vi "frameratetest_mono12.vi"() -> ()   [LabVIEW 2019]
panel:
  out "Software FPS":dbl
  out "Camera FPS":dbl
  out "Image":u16[][](graph)
  out "Camera Serial":string
  out "Camera Version":string
  out "Camera Model":string
  out "SMD":dbl
  in  "Scan Mode":dbl min=0.0 max=0.0
  in  "Exposure":dbl min=0.0 max=0.0
  out "EXP":dbl
  out "SVW":i32
  out "SHW":i32
  out "SVO":i32
  out "SHO":i32
  in  "V Width":i32 min=0 max=0
  in  "V Offset":i32 min=0 max=0
  in  "H Width":i32 min=0 max=0
  in  "H Offset":i32 min=0 max=0
  in  "Binning":u16(ring)=1 items=["1x1"=1, "2x2"=2, "4x4"=4]
  out "Elapsed Time":u32
  out "Total Frames":i32
  in  "Display":bool=TRUE
  out "error out":errorcluster
  in  "stop":bool
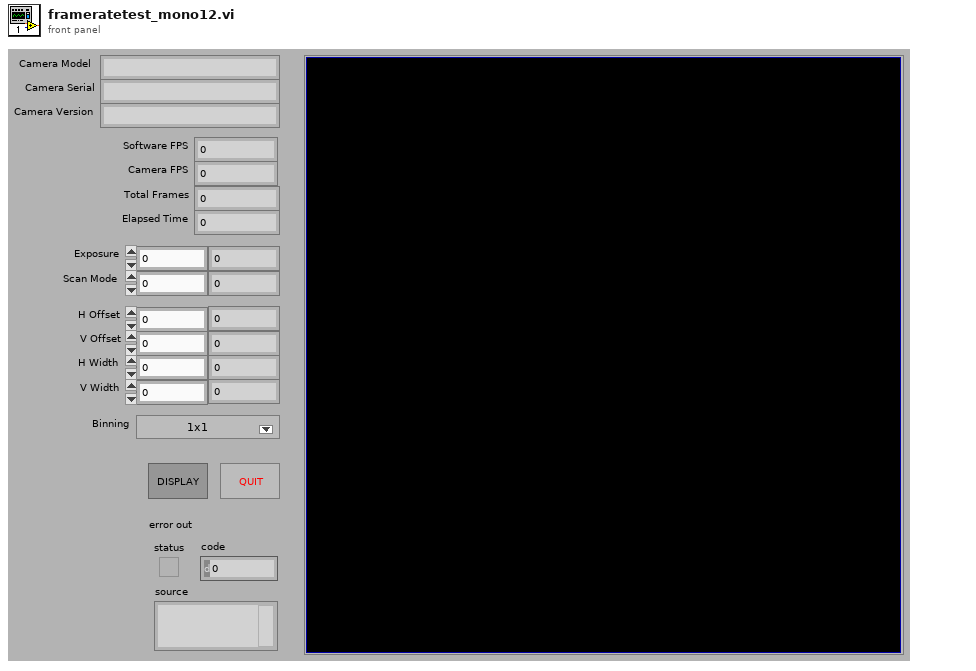
[diagram p1: front panel]
types:
  T1 = cluster{"Model":string, "Camera ID":string, "Firmware":string}
  T2 = typedef "LVMinMaxIncTypeDef.ctl" = cluster{"Minimum":dbl, "Maximum":dbl, "Increment":dbl}
  T3 = cluster{"H Offset":cluster{"Value":i32, "Limits":T2}, "V Offset":cluster{"Value":i32, "Limits":T2}, "H Size":cluster{"Value":i32, "Limits":T2}, "V Size":cluster{"Value":i32, "Limits":T2}}
  T4 = cluster{"H Offset":i32, "V Offset":i32, "H Width":i32, "V Width":i32}
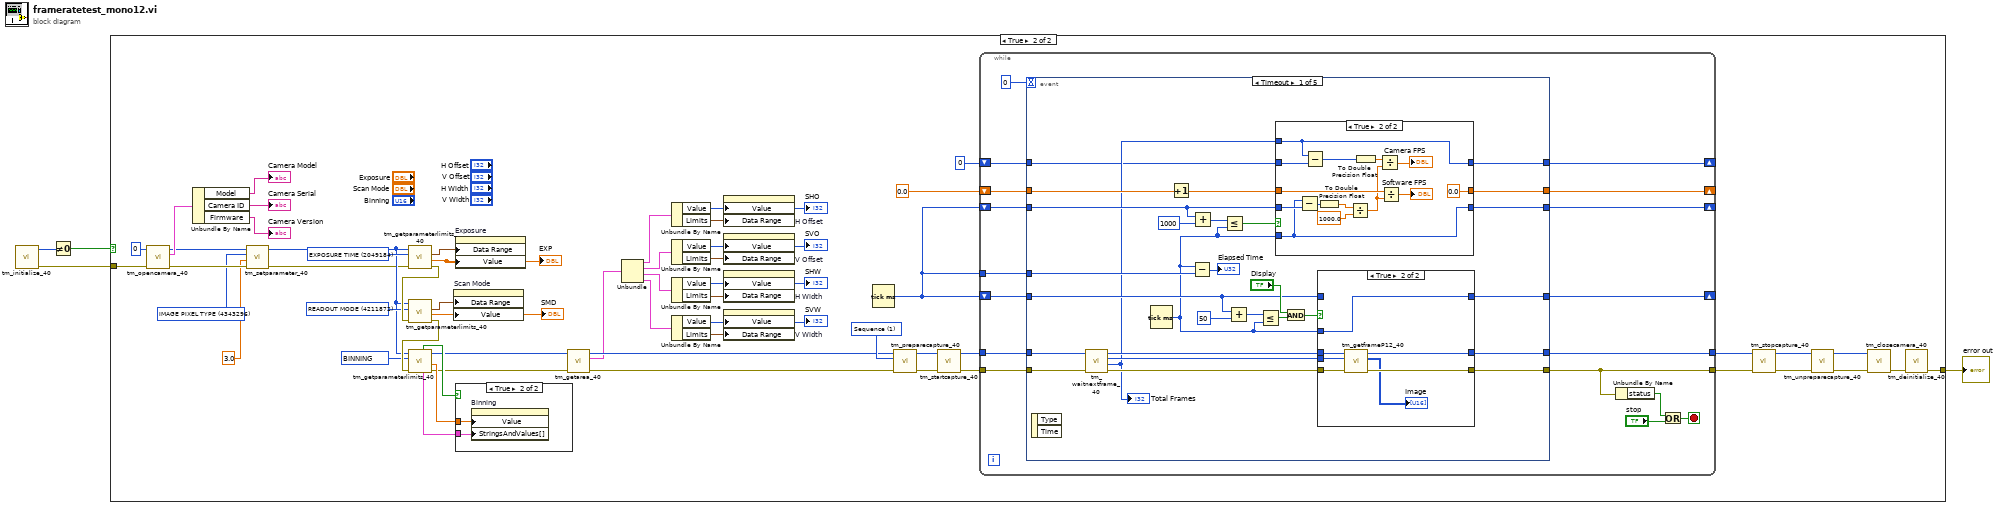
[diagram p0: block diagram]
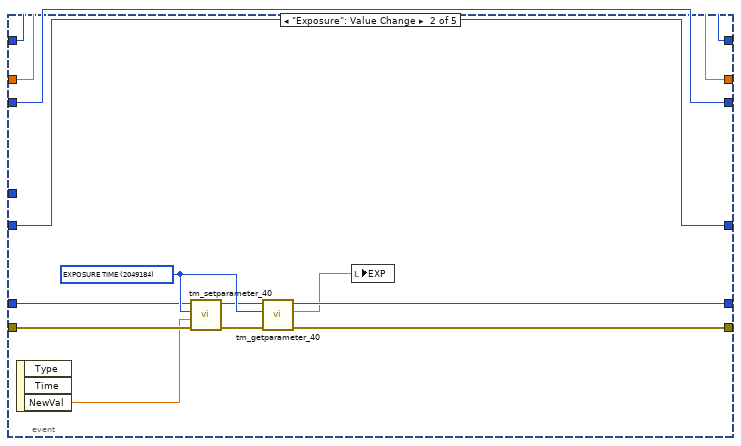
[diagram p6: hidden frame]
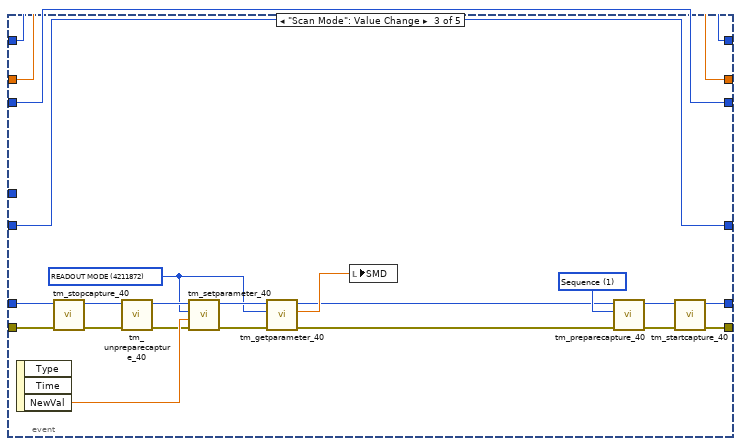
[diagram p7: hidden frame]
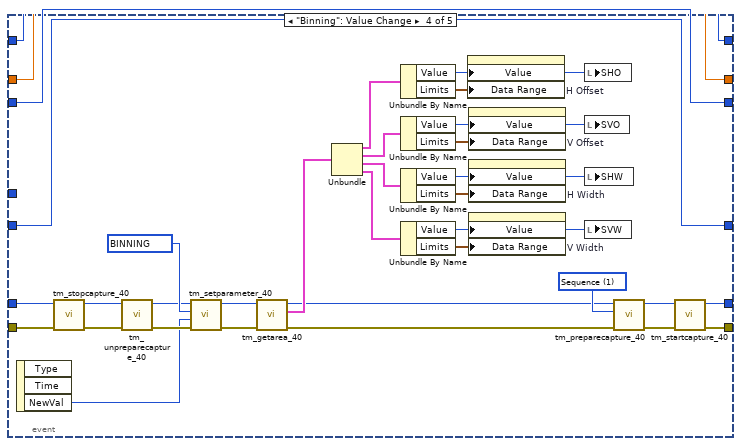
[diagram p8: hidden frame]
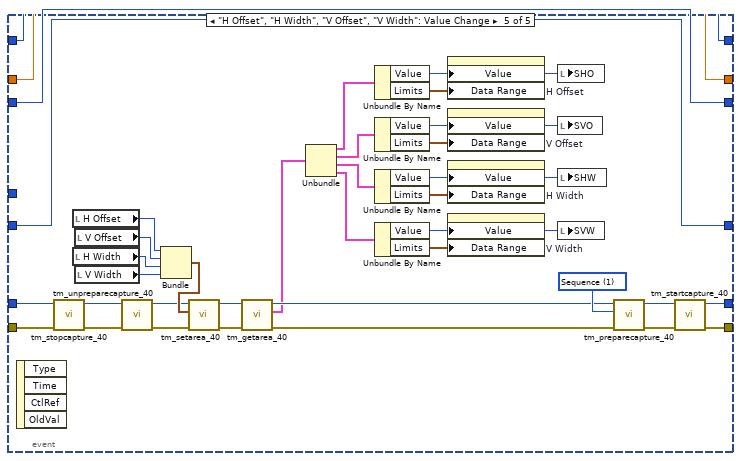
[diagram p9: hidden frame]
diagram:
  n1 = call <userlib>:"tm_initialize_40.vi"() -> ("error out"=w2:errorcluster, "Number Of Cameras"=w1:u32)  [unwired: 8 in, 2 out]
  n2 = Not Equal To 0?(x=w1) -> (x != 0?=w4:bool)
  n3 = case shown="True" w4 {
    tunnel: [w5 w59] -> w3
    tunnel: w2 -> [w5 w62]
    frame False {
    }
    frame True {
      w7 = u32 4343296 items=["SENSOR MODE"=4212128, "READOUT SPEED"=4211872, "READOUT DIRECTION"=4211904, "BIT PER CHANNEL"=4342976, "TRIGGER GLOBAL EXPOSURE"=2049680, "TRIGGER DELAY"=1066480, "INTERNAL TRIGGER HANDLING"=1066496, "SENSOR TEMPERATURE"=2115232, "SENSOR COOLER STATUS"=2115280, "EXPOSURE TIME"=2049184, "DEFECT CORRECT MODE"=4670368, "HOT PIXEL CORRECT LEVEL"=4670400, "BINNING"=4215968, "TIMING READOUT TIME"=4223904, "INTERNAL FRAME RATE"=4225952, "INTERNAL FRAME INTERVAL"=4225968, "INTERNAL LINE SPEED"=4226000, "INTERNAL LINE INTERVAL"=4226016, "IMAGE WIDTH"=4343200, "IMAGE HEIGHT"=4343216, "IMAGE ROWBYTES"=4343232, "IMAGE FRAMEBYTES"=4343248, "IMAGE PIXEL TYPE"=4343296, "NUMBER OF OUTPUT TRIGGER CONNECTOR"=1852320, "OUTPUT TRIGGER SOURCE[0]"=1852576, "OUTPUT TRIGGER SOURCE[1]"=1852832, "OUTPUT TRIGGER SOURCE[2]"=1853088, "OUTPUT TRIGGER POLARITY[0]"=1852592, "OUTPUT TRIGGER POLARITY[1]"=1852848, "OUTPUT TRIGGER POLARITY[2]"=1853104, "OUTPUT TRIGGER ACTIVE[0]"=1852608, "OUTPUT TRIGGER ACTIVE[1]"=1852864, "OUTPUT TRIGGER ACTIVE[2]"=1853120, "OUTPUT TRIGGER DELAY[0]"=1852624, "OUTPUT TRIGGER DELAY[1]"=1852880, "OUTPUT TRIGGER DELAY[2]"=1853136, "OUTPUT TRIGGER PERIOD[0]"=1852640, "OUTPUT TRIGGER PERIOD[1]"=1852896, "OUTPUT TRIGGER PERIOD[2]"=1853152, "OUTPUT TRIGGER KIND[0]"=1852656, "OUTPUT TRIGGER KIND[1]"=1852912, "OUTPUT TRIGGER KIND[2]"=1853168, "OUTPUT TRIGGER BASE SENSOR[0]"=1852672, "OUTPUT TRIGGER BASE SENSOR[1]"=1852928, "OUTPUT TRIGGER BASE SENSOR[2]"=1853184, "OUTPUT TRIGGER PRE HSYNC COUNT"=1852704] ("Parameter")
      w33 = u32 2049184 items=["BINNING"=4215968, "BITS PER CHANNEL"=4342976, "ACTIVE VIEW INDEX"=4343136, "CCD MODE"=4212384, "SENSOR MODE"=4212128, "READOUT MODE"=4211872, "EXPOSURE TIME"=2049184, "CONTRAST GAIN"=3163312, "CONTRAST OFFSET"=3163328, "LIGHT MODE"=2114720, "SENSITIVITY"=2114992, "WHITE BALANCE"=3163568, "PHOTON IMAGING MODE"=2115200, "HIGH DYNAMIC RANGE MODE"=3163360, "TRIGGER SOURCE"=1066144, "TRIGGER ACTIVE"=1066160, "TRIGGER MODE"=1066400, "TRIGGER POLARITY"=1066416, "TRIGGER GLOBAL EXPOSURE"=2049680, "FIRST TRIGGER BEHAVIOR"=2049696, "TRIGGER TIMES"=1066448, "OUTPUT TRIGGER POLARITY"=1852592, "OUTPUT TRIGGER DELAY"=1852624, "OUTPUT TRIGGER PERIOD"=1852640, "TEMPERATURE"=2115232, "TEMPERATURE TARGET"=2115264, "SENSOR COOLER FAN"=2115296, "MECHANICAL SHUTTER"=2115488, "BACK FOCUS POSITION"=8422304, "FRAMEBUNDLE MODE"=4346784, "FRAMEBUNDLE NUMBER"=4346800, "LINEBUNDLE HEIGHT"=4212192, "TRIGGER CONNECTOR"=1066432, "IMAGE PIXEL TYPE"=4343296, "OUTPUT TRIGGER KIND"=1852656, "READOUT DIRECTION"=4211904, "CHANNEL SYNC"=1852352] ("Parameter")
      w34 = u32 4211872 items=["BINNING"=4215968, "BITS PER CHANNEL"=4342976, "ACTIVE VIEW INDEX"=4343136, "CCD MODE"=4212384, "SENSOR MODE"=4212128, "READOUT MODE"=4211872, "EXPOSURE TIME"=2049184, "CONTRAST GAIN"=3163312, "CONTRAST OFFSET"=3163328, "LIGHT MODE"=2114720, "SENSITIVITY"=2114992, "WHITE BALANCE"=3163568, "PHOTON IMAGING MODE"=2115200, "HIGH DYNAMIC RANGE MODE"=3163360, "TRIGGER SOURCE"=1066144, "TRIGGER ACTIVE"=1066160, "TRIGGER MODE"=1066400, "TRIGGER POLARITY"=1066416, "TRIGGER GLOBAL EXPOSURE"=2049680, "FIRST TRIGGER BEHAVIOR"=2049696, "TRIGGER TIMES"=1066448, "OUTPUT TRIGGER POLARITY"=1852592, "OUTPUT TRIGGER DELAY"=1852624, "OUTPUT TRIGGER PERIOD"=1852640, "TEMPERATURE"=2115232, "TEMPERATURE TARGET"=2115264, "SENSOR COOLER FAN"=2115296, "MECHANICAL SHUTTER"=2115488, "BACK FOCUS POSITION"=8422304, "FRAMEBUNDLE MODE"=4346784, "FRAMEBUNDLE NUMBER"=4346800, "LINEBUNDLE HEIGHT"=4212192, "TRIGGER CONNECTOR"=1066432, "IMAGE PIXEL TYPE"=4343296, "OUTPUT TRIGGER KIND"=1852656, "READOUT DIRECTION"=4211904, "CHANNEL SYNC"=1852352] ("Parameter")
      w35 = u32 4215968 items=["BINNING"=4215968, "BITS PER CHANNEL"=4342976, "ACTIVE VIEW INDEX"=4343136, "CCD MODE"=4212384, "SENSOR MODE"=4212128, "READOUT MODE"=4211872, "EXPOSURE TIME"=2049184, "CONTRAST GAIN"=3163312, "CONTRAST OFFSET"=3163328, "LIGHT MODE"=2114720, "SENSITIVITY"=2114992, "WHITE BALANCE"=3163568, "PHOTON IMAGING MODE"=2115200, "HIGH DYNAMIC RANGE MODE"=3163360, "TRIGGER SOURCE"=1066144, "TRIGGER ACTIVE"=1066160, "TRIGGER MODE"=1066400, "TRIGGER POLARITY"=1066416, "TRIGGER GLOBAL EXPOSURE"=2049680, "FIRST TRIGGER BEHAVIOR"=2049696, "TRIGGER TIMES"=1066448, "OUTPUT TRIGGER POLARITY"=1852592, "OUTPUT TRIGGER DELAY"=1852624, "OUTPUT TRIGGER PERIOD"=1852640, "TEMPERATURE"=2115232, "TEMPERATURE TARGET"=2115264, "SENSOR COOLER FAN"=2115296, "MECHANICAL SHUTTER"=2115488, "BACK FOCUS POSITION"=8422304, "FRAMEBUNDLE MODE"=4346784, "FRAMEBUNDLE NUMBER"=4346800, "LINEBUNDLE HEIGHT"=4212192, "TRIGGER CONNECTOR"=1066432, "IMAGE PIXEL TYPE"=4343296, "OUTPUT TRIGGER KIND"=1852656, "READOUT DIRECTION"=4211904, "CHANNEL SYNC"=1852352] ("Parameter")
      w57 = 1 items=["Snap", "Sequence"] ("Capture mode")
      n4 = call <userlib>:"tm_opencamera_40.vi"("error in (no error)"=w62, "Camera Index"=u32 0) -> ("error out"=w11:errorcluster, "Camera Details"=w44:T1, "Handle out"=w10:u32)  [unwired: 7 in]
      n5 = Unbundle By Name(w44) -> ("Model"=→"Camera Model":string, "Camera ID"=→"Camera Serial":string, "Firmware"=→"Camera Version":string)
      n6 = call <userlib>:"tm_setparameter_40.vi"("error in (no error)"=w11, "Value in"=3.0, "Parameter"=w7, "Handle in"=w10) -> ("error out"=w8:errorcluster, "Handle out"=w9:u32)  [unwired: 6 in]
      n7 = call <userlib>:"tm_getparameterlimits_40.vi"("error in (no error)"=w8, "Parameter"=w33, "Handle in"=w9) -> ("error out"=w40:errorcluster, "default"=w25:dbl, "Range"=w26:cluster{"min":dbl, "max":dbl, "step":dbl})  [unwired: 2 in, 4 out]
      "EXP" <- w25
      n8 = call <userlib>:"tm_getparameterlimits_40.vi"("error in (no error)"=w40, "Parameter"=w34, "Handle in"=w9) -> ("error out"=w39:errorcluster, "default"=w27:dbl, "Range"=w28:cluster{"min":dbl, "max":dbl, "step":dbl})  [unwired: 2 in, 4 out]
      "SMD" <- w27
      n9 = call <userlib>:"tm_getparameterlimits_40.vi"("error in (no error)"=w39, "Parameter"=w35, "Handle in"=w9) -> ("error out"=w32:errorcluster, "default"=w37:dbl, "Handle out"=w31:u32, "Value Names"=w36:cluster{"Name":string, "Value":dbl}[], "Writable"=w38:bool)  [unwired: 2 in, 2 out]
      n10 = property on="Scan Mode" class="DigNum (strict)"("Data Range"=w28, "Value"=w27) -> ()  [unwired: 2 in, 2 out]
      n11 = property on="Exposure" class="DigNum (strict)"("Data Range"=w26, "Value"=w25) -> ()  [unwired: 2 in, 2 out]
      n12 = case shown="True" w38 {
        tunnel: w36 -> [_ w64]
        tunnel: w37 -> [_ w63]
        frame False {
        }
        frame True {
          n13 = property on="Binning" class="Ring (strict)"("Value"=w63, "StringsAndValues[]"=w64) -> ()  [unwired: 2 in, 2 out]
        }
      }
      n14 = call <userlib>:"tm_getarea_40.vi"("error in (no error)"=w32, "Handle in"=w31) -> ("error out"=w30:errorcluster, "Sub Region"=w20:T3, "Handle out"=w29:u32)  [unwired: 7 in]
      n15 = Unbundle(w20) -> ("H Offset"=w24:cluster{"Value":i32, "Limits":T2}, "V Offset"=w23:cluster{"Value":i32, "Limits":T2}, "H Size"=w22:cluster{"Value":i32, "Limits":T2}, "V Size"=w21:cluster{"Value":i32, "Limits":T2})
      n16 = Unbundle By Name(w24) -> ("Value"=w19:i32, "Limits"=w18:T2)
      "SHO" <- w19
      n17 = Unbundle By Name(w23) -> ("Value"=w13:i32, "Limits"=w12:T2)
      "SVO" <- w13
      n18 = Unbundle By Name(w22) -> ("Value"=w15:i32, "Limits"=w14:T2)
      "SHW" <- w15
      n19 = Unbundle By Name(w21) -> ("Value"=w17:i32, "Limits"=w16:T2)
      "SVW" <- w17
      n20 = property on="H Offset" class="DigNum (strict)"("Value"=w19, "Data Range"=w18) -> ()  [unwired: 2 in, 2 out]
      n21 = property on="V Offset" class="DigNum (strict)"("Value"=w13, "Data Range"=w12) -> ()  [unwired: 2 in, 2 out]
      n22 = property on="H Width" class="DigNum (strict)"("Value"=w15, "Data Range"=w14) -> ()  [unwired: 2 in, 2 out]
      n23 = property on="V Width" class="DigNum (strict)"("Value"=w17, "Data Range"=w16) -> ()  [unwired: 2 in, 2 out]
      n24 = Tick Count (ms)() -> (millisecond timer value=w52:u32)
      n25 = call <userlib>:"tm_preparecapture_40.vi"("error in (no error)"=w30, "Capture mode"=w57, "Handle in"=w29) -> ("error out"=w55:errorcluster, "Handle out"=w56:u32)  [unwired: 5 in, 2 out]
      n26 = call <userlib>:"tm_startcapture_40.vi"("error in (no error)"=w55, "Handle in"=w56) -> ("error out"=w54:errorcluster, "Handle out"=w53:u32)  [unwired: 8 in]
      n27 = while {
        tunnel: w54 -> [w71]
        tunnel: [w69] -> w51
        tunnel: [w68] -> w50
        shift-right: [w77] -> _
        shift-left: w52 -> [w75]
        shift-right: [w78] -> _
        shift-left: 0.0 -> [w76]
        shift-right: [w70] -> _
        shift-left: w52 -> [w73]
        tunnel: w53 -> [w72]
        tunnel: w52 -> [w74]
        shift-right: [w65] -> _
        shift-left: 0 -> [w66]
        stop <- w79 stop-if-true
        n28 = event shown="[0] Timeout" {
          selector: _ -> [_ _ _ _ _]
          dyn-events: _ -> [_ _ _ _ _]
          timeout: 0 -> [_ _ _ _ _]
          tunnel: [w86 w147 w169 w198 w235] -> w78
          tunnel: [w85 w148 w170 w199 w236] -> w77
          tunnel: w76 -> [w95 w147 w169 w198 w235]
          tunnel: w75 -> [w88 w148 w170 w199 w236]
          tunnel: w74 -> [w91 _ _ _ _]
          tunnel: w73 -> [w96 w149 w171 w205 w242]
          tunnel: w72 -> [w98 w142 w166 w197 w229]
          tunnel: w71 -> [w97 w144 w165 w196 w228]
          tunnel: [w94 w149 w171 w205 w242] -> w70
          tunnel: [w93 w139 w160 w200 w237] -> w69
          tunnel: [w92 w137 w161 w201 w238] -> w68
          tunnel: w66 -> [w83 w146 w159 w193 w223]
          tunnel: [w82 w146 w159 w193 w223] -> w65
          event Timeout {
            n29 = event-data() -> ()  [unwired: 1 in, 2 out]
            n30 = call <userlib>:"tm_waitnextframe_40.vi"("error in (no error)"=w97, "Handle in"=w98) -> ("error out"=w102:errorcluster, "Frame Count"=w84:i32, "Frame Index"=w101:i32, "Handle out"=w103:u32)  [unwired: 6 in]
            "Total Frames" <- w84
            n31 = Tick Count (ms)() -> (millisecond timer value=w90:u32)
            n32 = Increment(x=w95) -> (x+1=w87:dbl)
            n33 = Subtract(x=w90, y=w91) -> (x-y=→"Elapsed Time":u32)
            n34 = Add(x=w88, y=u32 1000) -> (x+y=w109:u32)
            n35 = Less Or Equal?(x=w109, y=w90) -> (x <= y?=w89:bool)
            n36 = Add(x=w96, y=u32 50) -> (x+y=w107:u32)
            n37 = Less Or Equal?(x=w107, y=w90) -> (x <= y?=w105:bool)
            n38 = case shown="True" w89 {
              tunnel: w88 -> [w112 w121]
              tunnel: [w112 w118] -> w85
              tunnel: w87 -> [w111 w124]
              tunnel: w90 -> [_ w118]
              tunnel: [w111 0.0] -> w86
              tunnel: w84 -> [_ w113]
              tunnel: w83 -> [w110 w116]
              tunnel: [w110 w113] -> w82
              frame False {
              }
              frame True {
                n39 = Subtract(x=w118, y=w121) -> (x-y=w120:u32)
                n40 = Subtract(x=w113, y=w116) -> (x-y=w114:i32)
                n41 = To Double Precision Float(number=w120) -> (double precision float=w126:dbl)
                n42 = Divide(x=w126, y=1000.0) -> (x/y=w117:dbl)
                n43 = To Double Precision Float(number=w114) -> (double precision float=w115:dbl)
                n44 = Divide(x=w115, y=w117) -> (x/y=→"Camera FPS":dbl)
                n45 = Divide(x=w124, y=w117) -> (x/y=→"Software FPS":dbl)
              }
            }
            n46 = And(x="Display", y=w105) -> (x .and. y?=w100:bool)
            n47 = case shown="True" w100 {
              tunnel: w96 -> [w129 _]
              tunnel: w90 -> [_ w136]
              tunnel: [w129 w136] -> w94
              tunnel: w103 -> [w128 w135]
              tunnel: w102 -> [w127 w134]
              tunnel: [w128 w133] -> w93
              tunnel: [w127 w132] -> w92
              tunnel: w101 -> [_ w130]
              frame False {
              }
              frame True {
                n48 = call <userlib>:"tm_getframeP12_40.vi"("error in (no error)"=w134, "Frame Index"=w130, "Handle in"=w135) -> ("error out"=w132:errorcluster, "Data"=→"Image":u16[][], "Handle out"=w133:u32)  [unwired: 5 in, 1 out]
              }
            }
          }
          event "Exposure": Value Change {
            w145 = u32 2049184 items=["SENSOR MODE"=4212128, "CCD MODE"=4212384, "READOUT MODE"=4211872, "ACTIVE VIEW INDEX"=4343136, "BITS PER CHANNEL"=4342976, "IMAGE PIXEL TYPE"=4343296, "BINNING"=4215968, "EXPOSURE TIME"=2049184, "CONTRAST GAIN"=3163312, "CONTRAST OFFSET"=3163328, "LIGHT MODE"=2114720, "SENSITIVITY"=2114992, "PHOTON IMAGING MODE"=2115200, "HIGH DYNAMIC RANGE MODE"=3163360, "WHITE BALANCE"=3163568, "TEMPERATURE"=2115232, "TEMPERATURE TARGET"=2115264, "SENSOR COOLER FAN"=2115296, "LINEBUNDLE HEIGHT"=4212192, "MECHANICAL SHUTTER"=2115488, "BACK FOCUS POSITION"=8422304, "TRIGGER CONNECTOR"=1066432, "TRIGGER SOURCE"=1066144, "OUTPUT TRIGGER SOURCE"=1852576, "TRIGGER GLOBAL EXPOSURE"=2049680, "FIRST TRIGGER BEHAVIOR"=2049696, "CHANNEL SYNC"=1852352, "READOUT DIRECTION"=4211904, "PRE HSYNC COUNT"=1852704] ("Parameter")
            n49 = event-data() -> ("NewVal"=w143:dbl)  [unwired: 1 in, 2 out]
            n50 = call <userlib>:"tm_setparameter_40.vi"("error in (no error)"=w144, "Value in"=w143, "Parameter"=w145, "Handle in"=w142) -> ("error out"=w141:errorcluster, "Handle out"=w140:u32)  [unwired: 6 in]
            n51 = call <userlib>:"tm_getparameter_40.vi"("error in (no error)"=w141, "Parameter"=w145, "Handle in"=w140) -> ("error out"=w137:errorcluster, "Value out"=w138:dbl, "Handle out"=w139:u32)  [unwired: 6 in]
            n52 = local write "EXP"(w138) -> ()
          }
          event "Scan Mode": Value Change {
            w150 = u32 4211872 items=["SENSOR MODE"=4212128, "CCD MODE"=4212384, "READOUT MODE"=4211872, "ACTIVE VIEW INDEX"=4343136, "BITS PER CHANNEL"=4342976, "IMAGE PIXEL TYPE"=4343296, "BINNING"=4215968, "EXPOSURE TIME"=2049184, "CONTRAST GAIN"=3163312, "CONTRAST OFFSET"=3163328, "LIGHT MODE"=2114720, "SENSITIVITY"=2114992, "PHOTON IMAGING MODE"=2115200, "HIGH DYNAMIC RANGE MODE"=3163360, "WHITE BALANCE"=3163568, "TEMPERATURE"=2115232, "TEMPERATURE TARGET"=2115264, "SENSOR COOLER FAN"=2115296, "LINEBUNDLE HEIGHT"=4212192, "MECHANICAL SHUTTER"=2115488, "BACK FOCUS POSITION"=8422304, "TRIGGER CONNECTOR"=1066432, "TRIGGER SOURCE"=1066144, "OUTPUT TRIGGER SOURCE"=1852576, "TRIGGER GLOBAL EXPOSURE"=2049680, "FIRST TRIGGER BEHAVIOR"=2049696, "CHANNEL SYNC"=1852352, "READOUT DIRECTION"=4211904, "PRE HSYNC COUNT"=1852704] ("Parameter")
            w164 = 1 items=["Snap", "Sequence"] ("Capture mode")
            n53 = event-data() -> ("NewVal"=w155:dbl)  [unwired: 1 in, 2 out]
            n54 = call <userlib>:"tm_stopcapture_40.vi"("error in (no error)"=w165, "Handle in"=w166) -> ("error out"=w167:errorcluster, "Handle out"=w168:u32)  [unwired: 8 in]
            n55 = call <userlib>:"tm_unpreparecapture_40.vi"("error in (no error)"=w167, "Handle in"=w168) -> ("error out"=w153:errorcluster, "Handle out"=w154:u32)  [unwired: 8 in]
            n56 = call <userlib>:"tm_setparameter_40.vi"("error in (no error)"=w153, "Value in"=w155, "Parameter"=w150, "Handle in"=w154) -> ("error out"=w152:errorcluster, "Handle out"=w151:u32)  [unwired: 6 in]
            n57 = call <userlib>:"tm_getparameter_40.vi"("error in (no error)"=w152, "Parameter"=w150, "Handle in"=w151) -> ("error out"=w158:errorcluster, "Value out"=w157:dbl, "Handle out"=w156:u32)  [unwired: 6 in]
            n58 = local write "SMD"(w157) -> ()
            n59 = call <userlib>:"tm_preparecapture_40.vi"("error in (no error)"=w158, "Capture mode"=w164, "Handle in"=w156) -> ("error out"=w162:errorcluster, "Handle out"=w163:u32)  [unwired: 5 in, 2 out]
            n60 = call <userlib>:"tm_startcapture_40.vi"("error in (no error)"=w162, "Handle in"=w163) -> ("error out"=w161:errorcluster, "Handle out"=w160:u32)  [unwired: 8 in]
          }
          event "Binning": Value Change {
            w191 = u32 4215968 items=["BINNING"=4215968, "BITS PER CHANNEL"=2, "ACTIVE VIEW INDEX"=3, "CCD MODE"=4, "SENSOR MODE"=5, "READOUT MODE"=6, "EXPOSURE TIME"=7, "CONTRAST GAIN"=8, "CONTRAST OFFSET"=9, "LIGHT MODE"=10, "SENSITIVITY"=11, "WHITE BALANCE"=12, "PHOTON IMAGING MODE"=13, "HIGH DYNAMIC RANGE MODE"=14, "TRIGGER SOURCE"=15, "TRIGGER ACTIVE"=16, "TRIGGER MODE"=17, "TRIGGER POLARITY"=18, "TRIGGER GLOBAL EXPOSURE"=19, "FIRST TRIGGER BEHAVIOR"=20, "TRIGGER TIMES"=21, "OUTPUT TRIGGER POLARITY"=22, "OUTPUT TRIGGER DELAY"=23, "OUTPUT TRIGGER PERIOD"=24, "TEMPERATURE"=25, "TEMPERATURE TARGET"=26, "SENSOR COOLER FAN"=27, "MECHANICAL SHUTTER"=28, "BACK FOCUS POSITION"=29, "FRAMEBUNDLE MODE"=30, "FRAMEBUNDLE NUMBER"=31, "LINEBUNDLE HEIGHT"=32, "TRIGGER CONNECTOR"=33, "IMAGE PIXEL TYPE"=34, "OUTPUT TRIGGER KIND"=35, "READOUT DIRECTION"=36, "CHANNEL SYNC"=37] ("Parameter")
            w204 = 1 items=["Snap", "Sequence"] ("Capture mode")
            n61 = event-data() -> ("NewVal"=w189:u16)  [unwired: 1 in, 2 out]
            n62 = call <userlib>:"tm_stopcapture_40.vi"("error in (no error)"=w196, "Handle in"=w197) -> ("error out"=w194:errorcluster, "Handle out"=w195:u32)  [unwired: 8 in]
            n63 = call <userlib>:"tm_unpreparecapture_40.vi"("error in (no error)"=w194, "Handle in"=w195) -> ("error out"=w192:errorcluster, "Handle out"=w190:u32)  [unwired: 8 in]
            n64 = call <userlib>:"tm_setparameter_40.vi"("error in (no error)"=w192, "Value in"=w189, "Parameter"=w191, "Handle in"=w190) -> ("error out"=w186:errorcluster, "Handle out"=w187:u32)  [unwired: 6 in]
            n65 = call <userlib>:"tm_getarea_40.vi"("error in (no error)"=w186, "Handle in"=w187) -> ("error out"=w184:errorcluster, "Sub Region"=w188:T3, "Handle out"=w185:u32)  [unwired: 7 in]
            n66 = Unbundle(w188) -> ("H Offset"=w175:cluster{"Value":i32, "Limits":T2}, "V Offset"=w174:cluster{"Value":i32, "Limits":T2}, "H Size"=w173:cluster{"Value":i32, "Limits":T2}, "V Size"=w172:cluster{"Value":i32, "Limits":T2})
            n67 = Unbundle By Name(w175) -> ("Value"=w183:i32, "Limits"=w182:T2)
            n68 = Unbundle By Name(w174) -> ("Value"=w181:i32, "Limits"=w180:T2)
            n69 = Unbundle By Name(w173) -> ("Value"=w179:i32, "Limits"=w178:T2)
            n70 = Unbundle By Name(w172) -> ("Value"=w177:i32, "Limits"=w176:T2)
            n71 = property on="H Offset" class="DigNum (strict)"("Value"=w183, "Data Range"=w182) -> ()  [unwired: 2 in, 2 out]
            n72 = property on="V Offset" class="DigNum (strict)"("Value"=w181, "Data Range"=w180) -> ()  [unwired: 2 in, 2 out]
            n73 = property on="H Width" class="DigNum (strict)"("Value"=w179, "Data Range"=w178) -> ()  [unwired: 2 in, 2 out]
            n74 = property on="V Width" class="DigNum (strict)"("Value"=w177, "Data Range"=w176) -> ()  [unwired: 2 in, 2 out]
            n75 = local write "SHO"(w183) -> ()
            n76 = local write "SVO"(w181) -> ()
            n77 = local write "SHW"(w179) -> ()
            n78 = local write "SVW"(w177) -> ()
            n79 = call <userlib>:"tm_preparecapture_40.vi"("error in (no error)"=w184, "Capture mode"=w204, "Handle in"=w185) -> ("error out"=w202:errorcluster, "Handle out"=w203:u32)  [unwired: 5 in, 2 out]
            n80 = call <userlib>:"tm_startcapture_40.vi"("error in (no error)"=w202, "Handle in"=w203) -> ("error out"=w201:errorcluster, "Handle out"=w200:u32)  [unwired: 8 in]
          }
          event "H Offset", "H Width", "V Offset", "V Width": Value Change {
            w241 = 1 items=["Snap", "Sequence"] ("Capture mode")
            n81 = event-data() -> ()  [unwired: 1 in, 4 out]
            n82 = call <userlib>:"tm_stopcapture_40.vi"("error in (no error)"=w228, "Handle in"=w229) -> ("error out"=w226:errorcluster, "Handle out"=w227:u32)  [unwired: 8 in]
            n83 = local read "H Offset"() -> (w232:i32)
            n84 = local read "H Width"() -> (w233:i32)
            n85 = local read "V Offset"() -> (w234:i32)
            n86 = local read "V Width"() -> (w231:i32)
            n87 = call <userlib>:"tm_unpreparecapture_40.vi"("error in (no error)"=w226, "Handle in"=w227) -> ("error out"=w224:errorcluster, "Handle out"=w225:u32)  [unwired: 8 in]
            n88 = Bundle("H Offset"=w232, "V Offset"=w234, "H Width"=w233, "V Width"=w231) -> (w230:T4)  [unwired: 1 in]
            n89 = call <userlib>:"tm_setarea_40.vi"("error in (no error)"=w224, "Sub Region"=w230, "Handle in"=w225) -> ("error out"=w221:errorcluster, "Handle out"=w222:u32)  [unwired: 7 in]
            n90 = call <userlib>:"tm_getarea_40.vi"("error in (no error)"=w221, "Handle in"=w222) -> ("error out"=w219:errorcluster, "Sub Region"=w211:T3, "Handle out"=w220:u32)  [unwired: 7 in]
            n91 = Unbundle(w211) -> ("H Offset"=w218:cluster{"Value":i32, "Limits":T2}, "V Offset"=w217:cluster{"Value":i32, "Limits":T2}, "H Size"=w216:cluster{"Value":i32, "Limits":T2}, "V Size"=w215:cluster{"Value":i32, "Limits":T2})
            n92 = Unbundle By Name(w218) -> ("Value"=w214:i32, "Limits"=w213:T2)
            n93 = Unbundle By Name(w217) -> ("Value"=w212:i32, "Limits"=w207:T2)
            n94 = Unbundle By Name(w216) -> ("Value"=w208:i32, "Limits"=w206:T2)
            n95 = Unbundle By Name(w215) -> ("Value"=w210:i32, "Limits"=w209:T2)
            n96 = property on="H Offset" class="DigNum (strict)"("Value"=w214, "Data Range"=w213) -> ()  [unwired: 2 in, 2 out]
            n97 = property on="V Offset" class="DigNum (strict)"("Value"=w212, "Data Range"=w207) -> ()  [unwired: 2 in, 2 out]
            n98 = property on="H Width" class="DigNum (strict)"("Value"=w208, "Data Range"=w206) -> ()  [unwired: 2 in, 2 out]
            n99 = property on="V Width" class="DigNum (strict)"("Value"=w210, "Data Range"=w209) -> ()  [unwired: 2 in, 2 out]
            n100 = local write "SHO"(w214) -> ()
            n101 = local write "SVO"(w212) -> ()
            n102 = local write "SHW"(w208) -> ()
            n103 = local write "SVW"(w210) -> ()
            n104 = call <userlib>:"tm_preparecapture_40.vi"("error in (no error)"=w219, "Capture mode"=w241, "Handle in"=w220) -> ("error out"=w239:errorcluster, "Handle out"=w240:u32)  [unwired: 5 in, 2 out]
            n105 = call <userlib>:"tm_startcapture_40.vi"("error in (no error)"=w239, "Handle in"=w240) -> ("error out"=w238:errorcluster, "Handle out"=w237:u32)  [unwired: 8 in]
          }
        }
        n106 = Unbundle By Name(w68) -> ("status"=w80:bool)
        n107 = Or(x=w80, y="stop") -> (x .or. y?=w79:bool)
      }
      n108 = call <userlib>:"tm_stopcapture_40.vi"("error in (no error)"=w50, "Handle in"=w51) -> ("error out"=w47:errorcluster, "Handle out"=w48:u32)  [unwired: 8 in]
      n109 = call <userlib>:"tm_unpreparecapture_40.vi"("error in (no error)"=w47, "Handle in"=w48) -> ("error out"=w46:errorcluster, "Handle out"=w49:u32)  [unwired: 8 in]
      n110 = call <userlib>:"tm_closecamera_40.vi"("error in (no error)"=w46, "Handle in"=w49) -> ("error out"=w60:errorcluster)  [unwired: 9 in]
      n111 = call <userlib>:"tm_deinitialize_40.vi"("error in (no error)"=w60) -> ("error out"=w59:errorcluster)  [unwired: 10 in]
    }
  }
  "error out" <- w3
